vi "Framework.Tx.vi"(8 "error in (no error)":errorcluster, 11 "Framework in":refnum<class "Framework.lvclass">) -> (0 "error out":errorcluster, 3 "Framework out":refnum<class "Framework.lvclass">)   [LabVIEW 2017, in "DSF Core.lvlib" / "Framework.lvclass"]
uses:
  Framework.lvclass
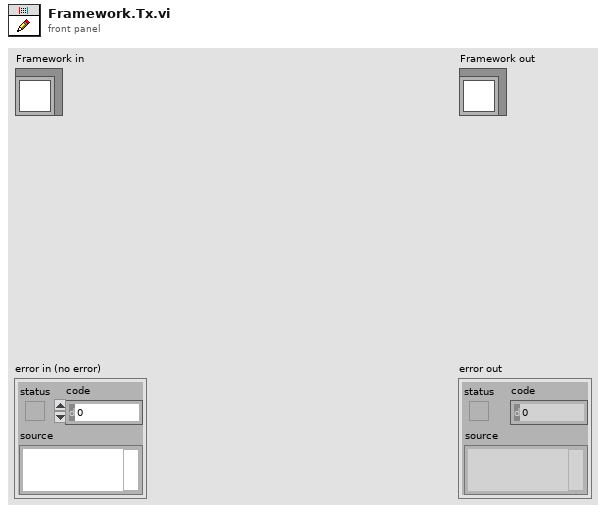
[diagram p1: front panel]
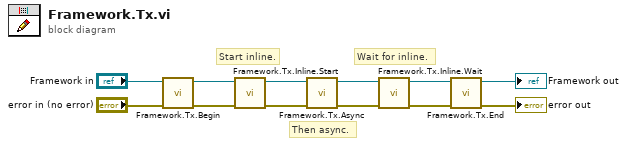
[diagram p0: block diagram]
diagram:
  # "Wait for inline."
  # "Start inline."
  # "Then async."
  n1 = call "Framework.Tx.Begin.vi"("error in (no error)"="error in (no error)", "Framework in"="Framework in") -> ("error out"=w5:errorcluster, "Framework out"=w6:refnum<class "Framework.lvclass">)  [unwired: 8 in]
  n2 = call "Framework.Tx.Inline.Start.vi"("error in (no error)"=w5, "Framework in"=w6) -> ("error out"=w10:errorcluster, "Framework out"=w9:refnum<class "Framework.lvclass">)  [unwired: 8 in]
  n3 = call "Framework.Tx.Async.vi"("error in (no error)"=w10, "Framework in"=w9) -> ("error out"=w12:errorcluster, "Framework out"=w11:refnum<class "Framework.lvclass">)  [unwired: 8 in]
  n4 = call "Framework.Tx.Inline.Wait.vi"("error in (no error)"=w12, "Framework in"=w11) -> ("error out"=w3:errorcluster, "Framework out"=w4:refnum<class "Framework.lvclass">)  [unwired: 8 in]
  n5 = call "Framework.Tx.End.vi"("error in (no error)"=w3, "Framework in"=w4) -> ("error out"=→"error out":errorcluster, "Framework out"=→"Framework out":refnum<class "Framework.lvclass">)  [unwired: 8 in]
